vi "Main.vi"   [LabVIEW 2024, in "PID Loop.lvlib" / "PID Loop.lvclass"]
uses:
  PID Loop.lvclass
  PID Loop.lvclass/PID Loop.ctl
types:
  T1 = typedef "PID Loop.lvlib/PID Loop.lvclass/Messages.ctl" = enum16{"Stop", "Start", "Exit", "Poll"}
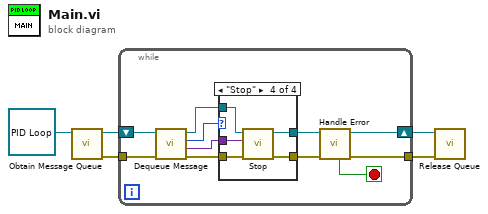
[diagram p0: block diagram]
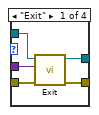
[diagram p2: hidden frame]
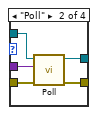
[diagram p3: hidden frame]
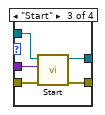
[diagram p4: hidden frame]
diagram:
  n1 = call-dynamic "Obtain Message Queue.vi"("PID Loop in"=refnum<class "PID Loop.lvclass"> refnum) -> ("error out"=w5:errorcluster, "PID Loop out"=w2:refnum<class "PID Loop.lvclass">)  [unwired: 9 in]
  n2 = while {
    tunnel: [w7] -> w4
    tunnel: w5 -> [w15]
    shift-right: [w9] -> w3
    shift-left: w2 -> [w11]
    stop <- w6 stop-if-true
    n3 = call-dynamic "Dequeue Message.vi"("error in (no error)"=w15, "PID Loop in"=w11) -> ("error out"=w16:errorcluster, "Data"=w13:variant, "Message"=w14:T1, "PID Loop out"=w12:refnum<class "PID Loop.lvclass">)  [unwired: 6 in]
    n4 = case shown="\"Stop\"" w14 {
      tunnel: [w18 w22 w28 w33] -> w8
      tunnel: w16 -> [w19 w25 w29 w34]
      tunnel: w13 -> [w17 w24 w30 w35]
      tunnel: w12 -> [w21 w26 w31 w36]
      tunnel: [w20 w23 w27 w32] -> w10
      frame "Exit" {
        n5 = call-dynamic "Exit.vi"("error in (no error)"=w19, "Data"=w17, "PID Loop in"=w21) -> ("error out"=w18:errorcluster, "PID Loop out"=w20:refnum<class "PID Loop.lvclass">)  [unwired: 7 in]
      }
      frame "Poll" {
        n6 = call "Poll.vi"("error in (no error)"=w25, "Data"=w24, "PID Loop in"=w26) -> ("error out"=w22:errorcluster, "PID Loop out"=w23:refnum<class "PID Loop.lvclass">)  [unwired: 7 in]
      }
      frame "Start" {
        n7 = call-dynamic "Start.vi"("error in (no error)"=w29, "Data"=w30, "PID Loop in"=w31) -> ("error out"=w28:errorcluster, "PID Loop out"=w27:refnum<class "PID Loop.lvclass">)  [unwired: 7 in]
      }
      frame "Stop" {
        n8 = call-dynamic "Stop.vi"("error in (no error)"=w34, "Data"=w35, "PID Loop in"=w36) -> ("error out"=w33:errorcluster, "PID Loop out"=w32:refnum<class "PID Loop.lvclass">)  [unwired: 7 in]
      }
    }
    n9 = call-dynamic "Handle Error.vi"("error in (no error)"=w8, "PID Loop in"=w10) -> ("error out"=w7:errorcluster, "PID Loop out"=w9:refnum<class "PID Loop.lvclass">, "Exit?"=w6:bool)  [unwired: 7 in]
  }
  n10 = call-dynamic "Release Queue.vi"("error in (no error)"=w4, "PID Loop in"=w3) -> ()  [unwired: 8 in, 2 out]
